vi "HandleRequest.vi"(11 "Web Request in":refnum<class "Web Request.lvclass">) -> (0 "error out":errorcluster, 3 "Web Request out":refnum<class "Web Request.lvclass">)   [LabVIEW 2014]
uses:
  <vilib>/wsapi/Web Request.lvclass
  Message.ctl
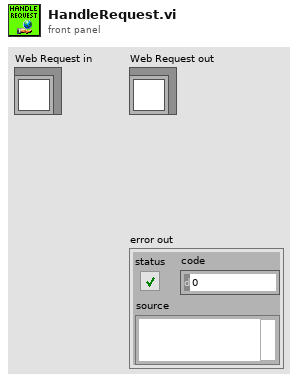
[diagram p1: front panel]
types:
  T1 = typedef "Message.ctl" = cluster{"Message":string, "Data":variant, "Response":refnum<queue>}
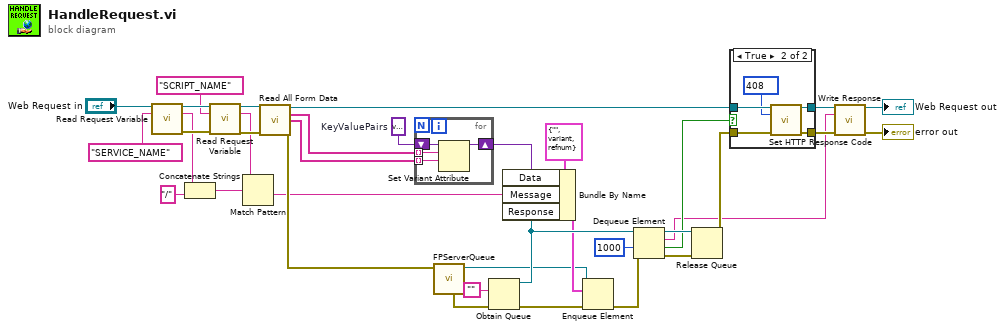
[diagram p0: block diagram]
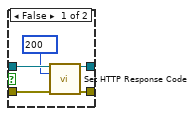
[diagram p2: hidden frame]
diagram:
  w21 = variant  # KeyValuePairs
  n1 = call <vilib>:"Read Request Variable.vi"("LabVIEW Web Service Request"="Web Request in", "variable name"="SERVICE_NAME") -> ("LabVIEW Web Service Request out"=w16:refnum<class "Web Request.lvclass">, "value"=w8:string, "error out"=w32:errorcluster)  [unwired: 11 in]
  n2 = Concatenate Strings(w8, "/" ("string")) -> (w9:string)
  n3 = call <vilib>:"Read Request Variable.vi"("LabVIEW Web Service Request"=w16, "variable name"="SCRIPT_NAME", "error in (no error)"=w32) -> ("LabVIEW Web Service Request out"=w14:refnum<class "Web Request.lvclass">, "value"=w10:string, "error out"=w33:errorcluster)  [unwired: 10 in]
  n4 = Match Pattern(string=w10, regular expression=w9) -> (after substring=w11:string)  [unwired: 1 in, 3 out]
  n5 = call <vilib>:"Read All Form Data.vi"("LabVIEW Web Service Request"=w14, "error in (no error)"=w33) -> ("LabVIEW Web Service Request out"=w3:refnum<class "Web Request.lvclass">, "Key"=w19:string[], "Value"=w20:string[], "error out"=w28:errorcluster)  [unwired: 9 in, 1 out]
  n6 = for {
    tunnel: w19 -> [w38] mode=indexing
    tunnel: w20 -> [w37] mode=indexing
    shift-right: [w39] -> w2
    shift-left: w21 -> [w40]
    n7 = Set Variant Attribute(Variant=w40, name=w38, value=w37) -> (Variant out=w39:variant)  [unwired: 1 in, 2 out]
  }
  n8 = call "FPServerQueue.vi"("error in (no error)"=w28) -> ("FPServer Queue"=w18:refnum<queue>, "error out"=w27:errorcluster)  [unwired: 9 in]
  n9 = Obtain Queue(element data type="", error in (no error)=w27) -> (queue out=w24:refnum<queue>, error out=w34:errorcluster)  [unwired: 3 in, 1 out]
  n10 = Bundle By Name(cluster=T1 {"Message"="", "Data"=variant, "Response"=refnum} ("Process Message"), "Data"=w2, "Message"=w11, "Response"=w24) -> (w23:T1)
  n11 = Enqueue Element(queue=w18, element=w23, error in (no error)=w34) -> (error out=w35:errorcluster)  [unwired: 1 in, 2 out]
  n12 = Dequeue Element(queue=w24, timeout in ms (-1)=1000, error in (no error)=w35) -> (queue out=w26:refnum<queue>, element=w5:string, timed out?=w7:bool, error out=w36:errorcluster)
  n13 = Release Queue(queue=w26, error in (no error)=w36) -> (error out=w31:errorcluster)  [unwired: 1 in, 2 out]
  n14 = case shown="True" w7 {
    tunnel: w3 -> [w42 w48]
    tunnel: [w43 w46] -> w6
    tunnel: w31 -> [w44 w50]
    tunnel: [w45 w49] -> w30
    frame False {
      w41 = 200 items=["100"=100, "101"=101, "200"=200, "201"=201, "202"=202, "203"=203, "204"=204, "205"=205, "206"=206, "300"=300, "301"=301, "302"=302, "303"=303, "304"=304, "305"=305, "306"=306, "307"=307, "400"=400, "401"=401, "402"=402, "403"=403, "404"=404, "405"=405, "406"=406, "407"=407, "408"=408, "409"=409, "410"=410, "411"=411, "412"=412, "413"=413, "414"=414, "415"=415, "416"=416, "417"=417, "500"=500, "501"=501, "502"=502, "503"=503, "504"=504, "505"=505] ("response code (200)")
      n15 = call <vilib>:"Set HTTP Response Code.vi"("LabVIEW Web Service Request"=w42, "response code (200)"=w41, "error in (no error)"=w44) -> ("LabVIEW Web Service Request out"=w43:refnum<class "Web Request.lvclass">, "error out"=w45:errorcluster)  [unwired: 11 in]
    }
    frame True {
      w47 = 408 items=["100"=100, "101"=101, "200"=200, "201"=201, "202"=202, "203"=203, "204"=204, "205"=205, "206"=206, "300"=300, "301"=301, "302"=302, "303"=303, "304"=304, "305"=305, "306"=306, "307"=307, "400"=400, "401"=401, "402"=402, "403"=403, "404"=404, "405"=405, "406"=406, "407"=407, "408"=408, "409"=409, "410"=410, "411"=411, "412"=412, "413"=413, "414"=414, "415"=415, "416"=416, "417"=417, "500"=500, "501"=501, "502"=502, "503"=503, "504"=504, "505"=505] ("response code (200)")
      n16 = call <vilib>:"Set HTTP Response Code.vi"("LabVIEW Web Service Request"=w48, "response code (200)"=w47, "error in (no error)"=w50) -> ("LabVIEW Web Service Request out"=w46:refnum<class "Web Request.lvclass">, "error out"=w49:errorcluster)  [unwired: 11 in]
    }
  }
  n17 = call <vilib>:"Write Response.vi"("LabVIEW Web Service Request"=w6, "response string"=w5, "error in (no error)"=w30) -> ("LabVIEW Web Service Request out"=→"Web Request out":refnum<class "Web Request.lvclass">, "error out"=→"error out":errorcluster)  [unwired: 11 in]
